vi "PulsoQuadrado.vi"() -> ()   [LabVIEW 2011]
panel:
  in  "offset":dbl(knob) scale=0.0..1.0
  in  "Numeric":i32
  out "?":dbl
  out "?":dbl
  in  "wide pulse(ms)":dbl(knob) scale=0.1..2.0
  in  "Volt (V)":dbl(knob) scale=0.0..9.8
  out "Waveform Graph":dbl[](graph)
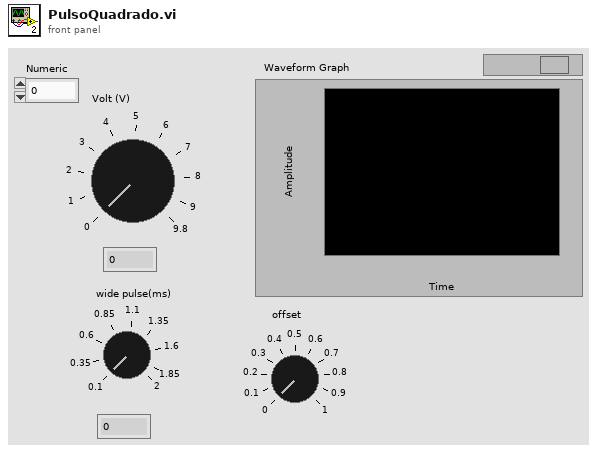
[diagram p1: front panel]
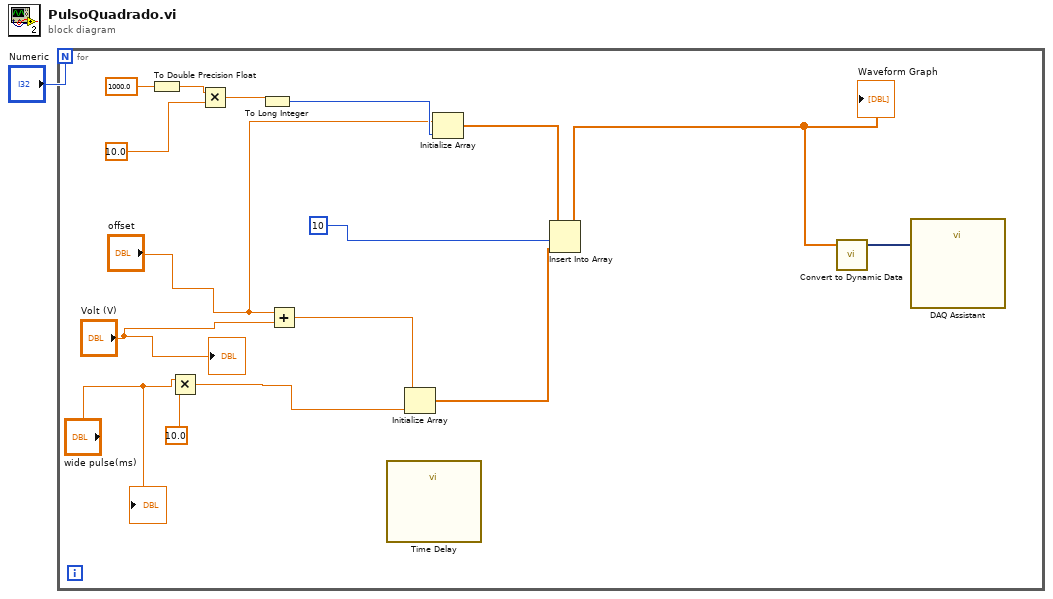
[diagram p0: block diagram]
diagram:
  n1 = for {
    N: "Numeric" -> [_]
    n2 = To Double Precision Float(number=1000.0) -> (double precision float=w14:dbl)
    n3 = Multiply(x="wide pulse(ms)", y=10.0) -> (x*y=w4:dbl)
    n4 = Multiply(x=w14, y=10.0) -> (x*y=w12:dbl)
    n5 = To Long Integer(number=w12) -> (32bit integer=w11:i32)
    n6 = Add(x="offset", y="Volt (V)") -> (x+y=w15:dbl)
    n7 = call "Time Delay"() -> ()  [unwired: 11 in, 1 out]
    n8 = Initialize Array(w15, w4) -> (w16:dbl[])
    n9 = Initialize Array("offset", w11) -> (w17:dbl[])
    n10 = Insert Into Array(array=w17, index=10, new element=w16) -> (w10:dbl[])
    "Waveform Graph" <- w10
    n11 = call "Convert to Dynamic Data"("Array"=w10) -> ("Dynamic Data Type"=w3:dynamicdata)  [unwired: 3 in]
    n12 = call "DAQ Assistant"("data"=w3) -> ()  [unwired: 16 in, 3 out]
    "?" <- "wide pulse(ms)"
    "?" <- "Volt (V)"
  }
